vi "OpenIVIsampleDMM.vi"(2 "measurement function (DC Volts)":i32=1, 3 "logical name (\"SampleDmm\")":string="SampleDmm") -> (0 "error out":errorcluster, 1 "instrument handle out":refnum<k15>="SampleDmm 3")   [LabVIEW 2013]
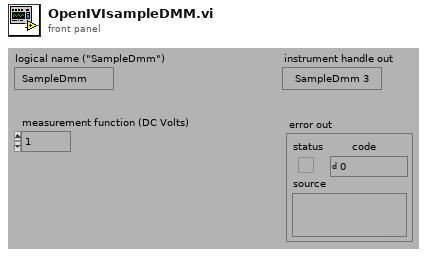
[diagram p1: front panel]
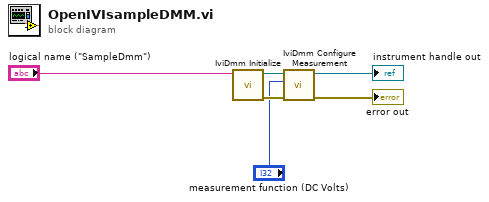
[diagram p0: block diagram]
diagram:
  n1 = call <vilib>:"IviDmm Initialize.vi"("logical name (\"SampleDmm\")"="logical name (\"SampleDmm\")") -> ("error out"=w3:errorcluster, "instrument handle out"=w2:refnum<k15>)  [unwired: 3 in, 6 out]
  n2 = call <vilib>:"IviDmm Configure Measurement.vi"("error in (no error)"=w3, "measurement function (DC Volts)"="measurement function (DC Volts)", "instrument handle"=w2) -> ("error out"=→"error out":errorcluster, "instrument handle out"=→"instrument handle out":refnum<k15>)  [unwired: 2 in, 5 out]
